vi "Configure Trigger (UDTV).vi"(6 "PGTHAN Time (2.6E-5)":dbl=2.6e-05, 7 "Horizontal Sync Time (1E-6)":dbl=1e-06, 8 "error in (no error)":errorcluster, 9 "Enable Horizontal Sync (F: Disable)":bool, 10 "Edge Number (1)":i32=1, 11 "VISA resource name":refnum<visa-resource-name>) -> (0 "error out":errorcluster, 3 "VISA resource name out":refnum<visa-resource-name>)   [LabVIEW 2017, in "Agilent 2000 3000 X-Series.lvlib"]
doc: "Configures the UDTV settings of the TV trigger mode. This VI is valid with the DSOX3VID extended Video triggering license.\n\nNote:\nThis VI is not supported by EDUX1052A/G, DSOX1202A/G, DSOX1204A/G models"
uses:
  Agilent 2000 3000 X-Series.lvlib
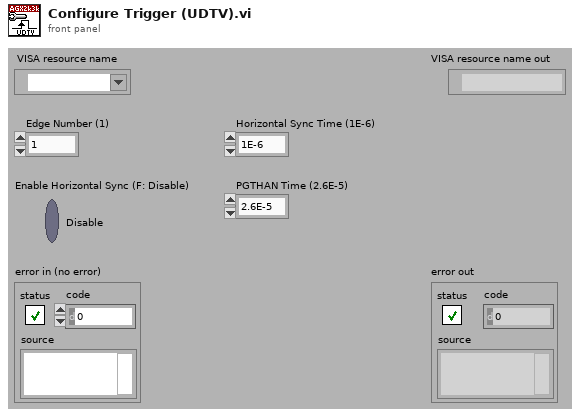
[diagram p1: front panel]
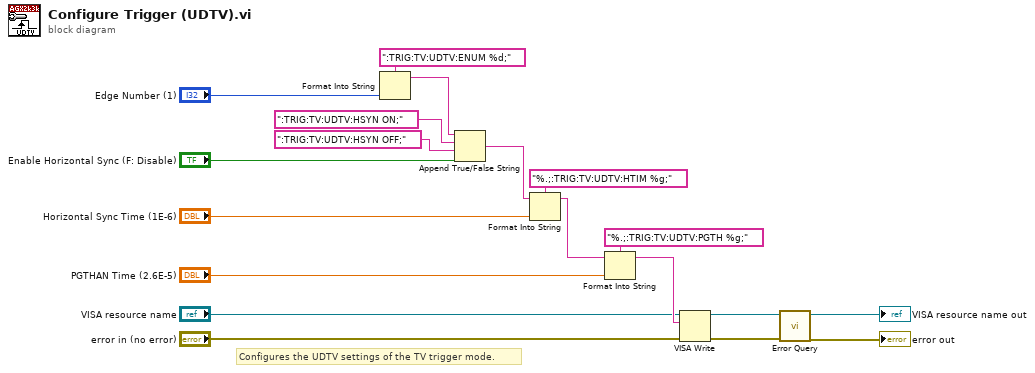
[diagram p0: block diagram]
diagram:
  # "Configures the UDTV settings of the TV trigger mode."
  n1 = Format Into String(format string=":TRIG:TV:UDTV:ENUM %d;", "Edge Number (1)") -> (resulting string=w17:string)  [unwired: 2 in, 1 out]
  n2 = Append True/False String(1:"Enable Horizontal Sync (F: Disable)", 2:":TRIG:TV:UDTV:HSYN OFF;", 3:":TRIG:TV:UDTV:HSYN ON;", 4:w17) -> (0:w13:string)
  n3 = Format Into String(format string="%.;:TRIG:TV:UDTV:HTIM %g;", initial string=w13, "Horizontal Sync Time (1E-6)") -> (resulting string=w10:string)  [unwired: 1 in, 1 out]
  n4 = Format Into String(format string="%.;:TRIG:TV:UDTV:PGTH %g;", initial string=w10, "PGTHAN Time (2.6E-5)") -> (resulting string=w7:string)  [unwired: 1 in, 1 out]
  n5 = VISA Write(VISA resource name="VISA resource name", write buffer=w7, error in (no error)="error in (no error)") -> (VISA resource name out=w4:refnum<visa-resource-name>, error out=w3:errorcluster)  [unwired: 1 out]
  n6 = call "Error Query.vi"("error in (no error)"=w3, "VISA resource name"=w4) -> ("error out"=→"error out":errorcluster, "VISA resource name out"=→"VISA resource name out":refnum<visa-resource-name>)  [unwired: 8 out]
